vi "Keyboard Input with Sensitivity Support.vi"(2 "device ID":refnum<k1>, 3 "Previous Control Cluster":T1 {"Yaw Speed" scale=-1.0..1.0; "Vertical Speed" scale=-1.0..1.0; "Pitch" scale=-1.0..1.0; "Roll" scale=-1.0..1.0}, 4 "Speed step":dbl, 5 "error in (no error)":errorcluster) -> (0 "error out":errorcluster, 1 "Control Cluster":T2 {"Roll" scale=-1.0..1.0; "Pitch" scale=-1.0..1.0; "Vertical Speed" scale=-1.0..1.0; "Yaw Speed" scale=-1.0..1.0})   [LabVIEW 2014]
uses:
  <vilib>/Utility/inputDevices.llb/keyboardAcquire.vi
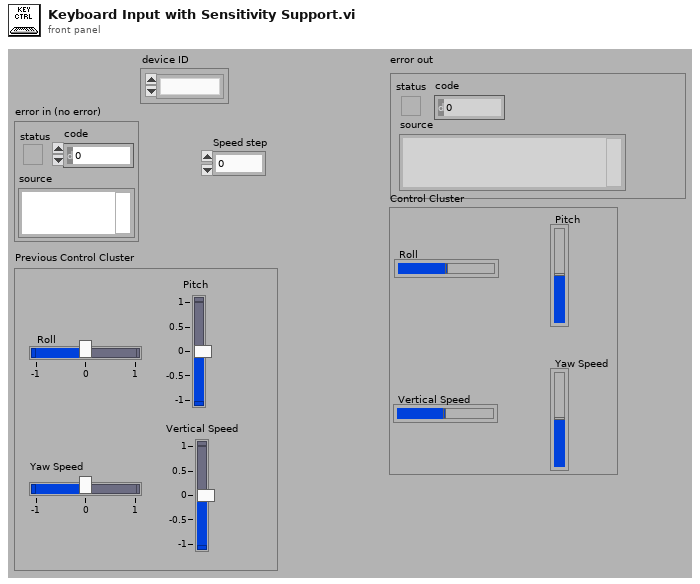
[diagram p1: front panel]
types:
  T1 = cluster{"Roll":sgl, "Pitch":sgl, "Vertical Speed":sgl, "Yaw Speed":sgl}
  T2 = cluster{"Roll":dbl, "Pitch":dbl, "Vertical Speed":dbl, "Yaw Speed":dbl}
  T3 = enum16{"0", "1", "2", "3", "4", "5", "6", "7", "8", "9", "A", "B", "C", "D", "E", "F", "G", "H", "I", "J", "K", "L", "M", "N", "O", "P", "Q", "R", "S", "T", "U", "V", "W", "X", "Y", "Z", "F1", "F2", "F3", "F4", "F5", "F6", "F7", "F8", "F9", "F10", "F11", "F12", "F13", "F14", "F15", "ADD", "BACK", "BACKSLASH", "CAPITAL", "COMMA", "DECIMAL", "DELETE", "DIVIDE", "DOWN", "END", "EQUALS", "ESCAPE", "GRAVE (`)", "HOME", "INSERT", "LBRACKET", "LCONTROL", "LEFT", "L ALT", "LSHIFT", "LWIN", "MINUS", "MULTIPLY", "NEXT", "NUMLOCK", "NUMPAD_0", "NUMPAD_1", "NUMPAD_2", "NUMPAD_3", "NUMPAD_4", "NUMPAD_5", "NUMPAD_6", "NUMPAD_7", "NUMPAD_8", "NUMPAD_9", "PAUSE", "PERIOD", "PRIOR (PG UP)", "RBRACKET", "RCONTROL", "RETURN", "RIGHT", "R ALT", "RSHIFT", "RWIN", "SCROLL", "SEMICOLON", "SLASH", "SPACE", "SUBTRACT", "TAB", "UP", "ENTER (num pad)", "' (quote)"}[]
  T4 = enum16{"0", "1", "2", "3", "4", "5", "6", "7", "8", "9", "A", "B", "C", "D", "E", "F", "G", "H", "I", "J", "K", "L", "M", "N", "O", "P", "Q", "R", "S", "T", "U", "V", "W", "X", "Y", "Z", "F1", "F2", "F3", "F4", "F5", "F6", "F7", "F8", "F9", "F10", "F11", "F12", "F13", "F14", "F15", "ADD", "BACK", "BACKSLASH", "CAPITAL", "COMMA", "DECIMAL", "DELETE", "DIVIDE", "DOWN", "END", "EQUALS", "ESCAPE", "GRAVE (`)", "HOME", "INSERT", "LBRACKET", "LCONTROL", "LEFT", "L ALT", "LSHIFT", "LWIN", "MINUS", "MULTIPLY", "NEXT", "NUMLOCK", "NUMPAD_0", "NUMPAD_1", "NUMPAD_2", "NUMPAD_3", "NUMPAD_4", "NUMPAD_5", "NUMPAD_6", "NUMPAD_7", "NUMPAD_8", "NUMPAD_9", "PAUSE", "PERIOD", "PRIOR (PG UP)", "RBRACKET", "RCONTROL", "RETURN", "RIGHT", "R ALT", "RSHIFT", "RWIN", "SCROLL", "SEMICOLON", "SLASH", "SPACE", "SUBTRACT", "TAB", "UP", "ENTER (num pad)", "' (quote)"}
  T5 = cluster{dbl, dbl, "New Speed":dbl, "New Speed":dbl}
  T6 = cluster{dbl, "New Speed":dbl, "New Speed":dbl, dbl}
  T7 = cluster{"New Speed":dbl, dbl, "New Speed":dbl, dbl}
  T8 = cluster{dbl, "New Speed":dbl, dbl, "New Speed":dbl}
  T9 = cluster{"New Speed":dbl, dbl, dbl, "New Speed":dbl}
  T10 = cluster{"New Speed":dbl, "New Speed":dbl, dbl, dbl}
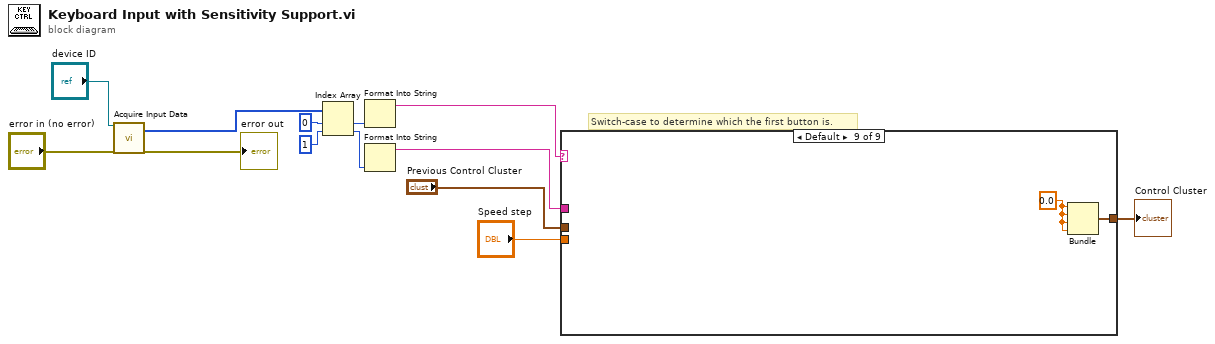
[diagram p0: block diagram]
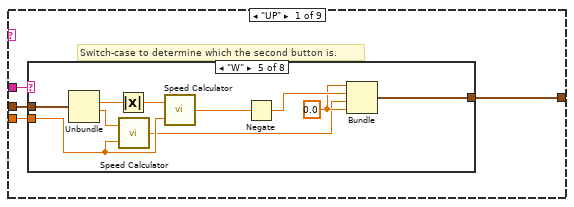
[diagram p2: hidden frame]
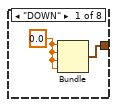
[diagram p3: hidden frame]
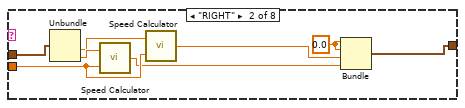
[diagram p4: hidden frame]
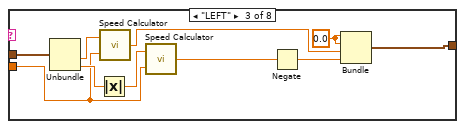
[diagram p5: hidden frame]
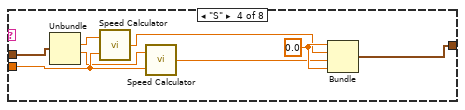
[diagram p6: hidden frame]
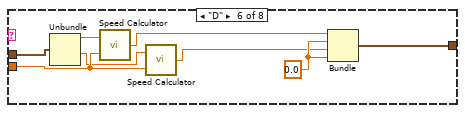
[diagram p7: hidden frame]
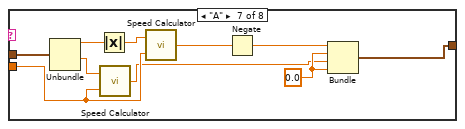
[diagram p8: hidden frame]
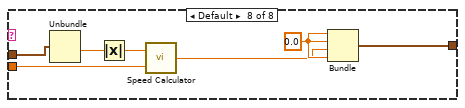
[diagram p9: hidden frame]
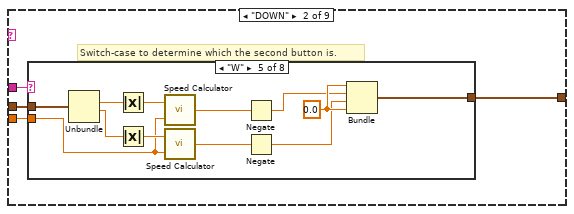
[diagram p10: hidden frame]
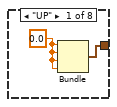
[diagram p11: hidden frame]
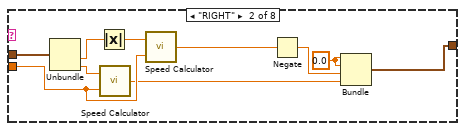
[diagram p12: hidden frame]
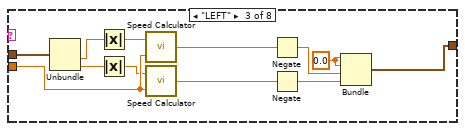
[diagram p13: hidden frame]
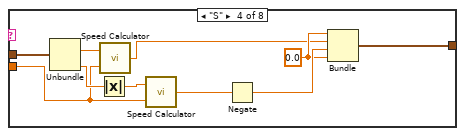
[diagram p14: hidden frame]
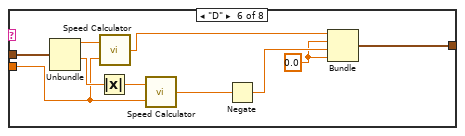
[diagram p15: hidden frame]
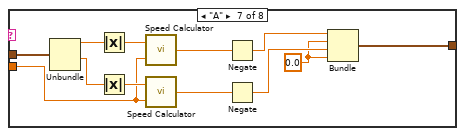
[diagram p16: hidden frame]
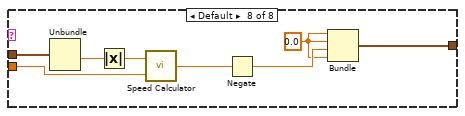
[diagram p17: hidden frame]
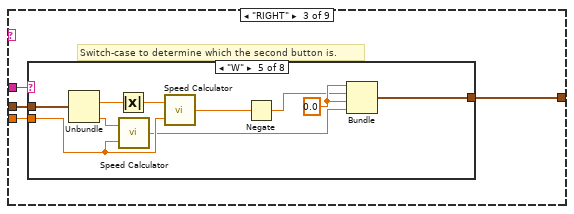
[diagram p18: hidden frame]
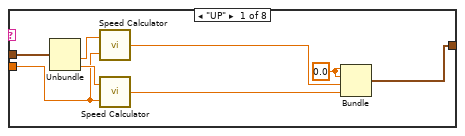
[diagram p19: hidden frame]
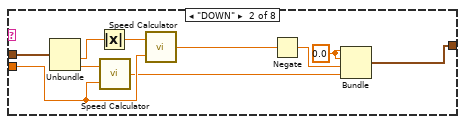
[diagram p20: hidden frame]
diagram:
  # "Switch-case to determine which the first button is."
  n1 = call-poly <vilib>:"Acquire Input Data.vi"("device ID"="device ID", "error in (no error)"="error in (no error)") -> ("keys pressed"=w7:T3, "error out"=→"error out":errorcluster)  [unwired: 15 in, 1 out]
  n2 = Index Array(array=w7, index #1=0, index #2=1) -> (element #1=w11:T4, element #2=w5:T4)
  n3 = Format Into String(w11) -> (resulting string=w13:string)  [unwired: 3 in, 1 out]
  n4 = Format Into String(w5) -> (resulting string=w4:string)  [unwired: 3 in, 1 out]
  n5 = case shown="Default" w13 {
    tunnel: w4 -> [w17 w83 w163 w230 w309 w375 w455 w521 _]
    tunnel: [w16 w82 w162 w228 w308 w374 w454 w520 w599] -> w2
    tunnel: "Speed step" -> [w15 w84 w164 w229 w310 w376 w456 w522 _]
    tunnel: "Previous Control Cluster" -> [w14 w81 w161 w227 w307 w373 w453 w519 _]
    frame "UP" {
      # "Switch-case to determine which the second button is."
      n6 = case shown="\"W\"" w17 {
        tunnel: [w18 w26 w37 w45 w55 w63 w73 w79] -> w16
        tunnel: w15 -> [_ w22 w31 w42 w49 w59 w68 w78]
        tunnel: w14 -> [_ w25 w34 w43 w52 w61 w70 w76]
        frame "DOWN" {
          w19 = 0.0
          n7 = Bundle(w19, w19, w19, w19) -> (w18:cluster{dbl, dbl, dbl, dbl})  [unwired: 1 in]
        }
        frame "RIGHT" {
          w27 = 0.0
          n8 = Unbundle(w25) -> ("Vertical Speed"=w20:sgl, "Yaw Speed"=w23:sgl)  [unwired: 2 out]
          n9 = call "Speed Calculator.vi"("Speed step"=w22, "Previous Speed"=w23) -> ("New Speed"=w21:dbl)
          n10 = call "Speed Calculator.vi"("Speed step"=w22, "Previous Speed"=w20) -> ("New Speed"=w24:dbl)
          n11 = Bundle(w27, w27, "New Speed"=w24, "New Speed"=w21) -> (w26:T5)  [unwired: 1 in]
        }
        frame "LEFT" {
          w35 = 0.0
          n12 = Unbundle(w34) -> ("Vertical Speed"=w30:sgl, "Yaw Speed"=w33:sgl)  [unwired: 2 out]
          n13 = Absolute Value(x=w33) -> (abs(x)=w32:sgl)
          n14 = call "Speed Calculator.vi"("Speed step"=w31, "Previous Speed"=w30) -> ("New Speed"=w29:dbl)
          n15 = call "Speed Calculator.vi"("Speed step"=w31, "Previous Speed"=w32) -> ("New Speed"=w28:dbl)
          n16 = Negate(x=w28) -> (-x=w36:dbl)
          n17 = Bundle(w35, w35, "New Speed"=w29, w36) -> (w37:cluster{dbl, dbl, "New Speed":dbl, dbl})  [unwired: 1 in]
        }
        frame "S" {
          w44 = 0.0
          n18 = Unbundle(w43) -> ("Pitch"=w38:sgl, "Vertical Speed"=w41:sgl)  [unwired: 2 out]
          n19 = call "Speed Calculator.vi"("Speed step"=w42, "Previous Speed"=w38) -> ("New Speed"=w39:dbl)
          n20 = call "Speed Calculator.vi"("Speed step"=w42, "Previous Speed"=w41) -> ("New Speed"=w40:dbl)
          n21 = Bundle(w44, "New Speed"=w39, "New Speed"=w40, w44) -> (w45:T6)  [unwired: 1 in]
        }
        frame "W" {
          w53 = 0.0
          n22 = Unbundle(w52) -> ("Pitch"=w51:sgl, "Vertical Speed"=w48:sgl)  [unwired: 2 out]
          n23 = Absolute Value(x=w51) -> (abs(x)=w50:sgl)
          n24 = call "Speed Calculator.vi"("Speed step"=w49, "Previous Speed"=w48) -> ("New Speed"=w47:dbl)
          n25 = call "Speed Calculator.vi"("Speed step"=w49, "Previous Speed"=w50) -> ("New Speed"=w46:dbl)
          n26 = Negate(x=w46) -> (-x=w54:dbl)
          n27 = Bundle(w53, w54, "New Speed"=w47, w53) -> (w55:cluster{dbl, dbl, "New Speed":dbl, dbl})  [unwired: 1 in]
        }
        frame "D" {
          w62 = 0.0
          n28 = Unbundle(w61) -> ("Roll"=w60:sgl, "Vertical Speed"=w58:sgl)  [unwired: 2 out]
          n29 = call "Speed Calculator.vi"("Speed step"=w59, "Previous Speed"=w60) -> ("New Speed"=w56:dbl)
          n30 = call "Speed Calculator.vi"("Speed step"=w59, "Previous Speed"=w58) -> ("New Speed"=w57:dbl)
          n31 = Bundle("New Speed"=w56, w62, "New Speed"=w57, w62) -> (w63:T7)  [unwired: 1 in]
        }
        frame "A" {
          w71 = 0.0
          n32 = Unbundle(w70) -> ("Roll"=w66:sgl, "Vertical Speed"=w69:sgl)  [unwired: 2 out]
          n33 = Absolute Value(x=w66) -> (abs(x)=w67:sgl)
          n34 = call "Speed Calculator.vi"("Speed step"=w68, "Previous Speed"=w69) -> ("New Speed"=w64:dbl)
          n35 = call "Speed Calculator.vi"("Speed step"=w68, "Previous Speed"=w67) -> ("New Speed"=w65:dbl)
          n36 = Negate(x=w65) -> (-x=w72:dbl)
          n37 = Bundle(w72, w71, "New Speed"=w64, w71) -> (w73:cluster{dbl, dbl, "New Speed":dbl, dbl})  [unwired: 1 in]
        }
        frame Default {
          w80 = 0.0
          n38 = Unbundle(w76) -> ("Vertical Speed"=w75:sgl)  [unwired: 3 out]
          n39 = Absolute Value(x=w75) -> (abs(x)=w74:sgl)
          n40 = call "Speed Calculator.vi"("Speed step"=w78, "Previous Speed"=w74) -> ("New Speed"=w77:dbl)
          n41 = Bundle(w80, w80, "New Speed"=w77, w80) -> (w79:cluster{dbl, dbl, "New Speed":dbl, dbl})  [unwired: 1 in]
        }
      }
    }
    frame "DOWN" {
      # "Switch-case to determine which the second button is."
      n42 = case shown="\"W\"" w83 {
        tunnel: [w86 w95 w108 w117 w130 w139 w152 w158] -> w82
        tunnel: w84 -> [_ w90 w103 w112 w123 w133 w141 w154]
        tunnel: w81 -> [_ w93 w106 w115 w128 w137 w148 w157]
        frame "UP" {
          w85 = 0.0
          n43 = Bundle(w85, w85, w85, w85) -> (w86:cluster{dbl, dbl, dbl, dbl})  [unwired: 1 in]
        }
        frame "RIGHT" {
          w94 = 0.0
          n44 = Unbundle(w93) -> ("Vertical Speed"=w92:sgl, "Yaw Speed"=w89:sgl)  [unwired: 2 out]
          n45 = Absolute Value(x=w92) -> (abs(x)=w91:sgl)
          n46 = call "Speed Calculator.vi"("Speed step"=w90, "Previous Speed"=w89) -> ("New Speed"=w88:dbl)
          n47 = call "Speed Calculator.vi"("Speed step"=w90, "Previous Speed"=w91) -> ("New Speed"=w87:dbl)
          n48 = Negate(x=w87) -> (-x=w96:dbl)
          n49 = Bundle(w94, w94, w96, "New Speed"=w88) -> (w95:cluster{dbl, dbl, dbl, "New Speed":dbl})  [unwired: 1 in]
        }
        frame "LEFT" {
          w107 = 0.0
          n50 = Unbundle(w106) -> ("Vertical Speed"=w105:sgl, "Yaw Speed"=w101:sgl)  [unwired: 2 out]
          n51 = Absolute Value(x=w105) -> (abs(x)=w104:sgl)
          n52 = Absolute Value(x=w101) -> (abs(x)=w102:sgl)
          n53 = call "Speed Calculator.vi"("Speed step"=w103, "Previous Speed"=w104) -> ("New Speed"=w100:dbl)
          n54 = call "Speed Calculator.vi"("Speed step"=w103, "Previous Speed"=w102) -> ("New Speed"=w99:dbl)
          n55 = Negate(x=w100) -> (-x=w98:dbl)
          n56 = Negate(x=w99) -> (-x=w97:dbl)
          n57 = Bundle(w107, w107, w98, w97) -> (w108:cluster{dbl, dbl, dbl, dbl})  [unwired: 1 in]
        }
        frame "S" {
          w116 = 0.0
          n58 = Unbundle(w115) -> ("Pitch"=w111:sgl, "Yaw Speed"=w114:sgl)  [unwired: 2 out]
          n59 = Absolute Value(x=w114) -> (abs(x)=w113:sgl)
          n60 = call "Speed Calculator.vi"("Speed step"=w112, "Previous Speed"=w111) -> ("New Speed"=w110:dbl)
          n61 = call "Speed Calculator.vi"("Speed step"=w112, "Previous Speed"=w113) -> ("New Speed"=w109:dbl)
          n62 = Negate(x=w109) -> (-x=w118:dbl)
          n63 = Bundle(w116, "New Speed"=w110, w118, w116) -> (w117:cluster{dbl, "New Speed":dbl, dbl, dbl})  [unwired: 1 in]
        }
        frame "W" {
          w129 = 0.0
          n64 = Unbundle(w128) -> ("Pitch"=w127:sgl, "Vertical Speed"=w125:sgl)  [unwired: 2 out]
          n65 = Absolute Value(x=w127) -> (abs(x)=w126:sgl)
          n66 = Absolute Value(x=w125) -> (abs(x)=w124:sgl)
          n67 = call "Speed Calculator.vi"("Speed step"=w123, "Previous Speed"=w126) -> ("New Speed"=w122:dbl)
          n68 = call "Speed Calculator.vi"("Speed step"=w123, "Previous Speed"=w124) -> ("New Speed"=w121:dbl)
          n69 = Negate(x=w122) -> (-x=w120:dbl)
          n70 = Negate(x=w121) -> (-x=w119:dbl)
          n71 = Bundle(w129, w120, w119, w129) -> (w130:cluster{dbl, dbl, dbl, dbl})  [unwired: 1 in]
        }
        frame "D" {
          w138 = 0.0
          n72 = Unbundle(w137) -> ("Roll"=w131:sgl, "Vertical Speed"=w136:sgl)  [unwired: 2 out]
          n73 = Absolute Value(x=w136) -> (abs(x)=w135:sgl)
          n74 = call "Speed Calculator.vi"("Speed step"=w133, "Previous Speed"=w131) -> ("New Speed"=w132:dbl)
          n75 = call "Speed Calculator.vi"("Speed step"=w133, "Previous Speed"=w135) -> ("New Speed"=w134:dbl)
          n76 = Negate(x=w134) -> (-x=w140:dbl)
          n77 = Bundle("New Speed"=w132, w138, w140, w138) -> (w139:cluster{"New Speed":dbl, dbl, dbl, dbl})  [unwired: 1 in]
        }
        frame "A" {
          w150 = 0.0
          n78 = Unbundle(w148) -> ("Roll"=w147:sgl, "Vertical Speed"=w145:sgl)  [unwired: 2 out]
          n79 = Absolute Value(x=w147) -> (abs(x)=w146:sgl)
          n80 = Absolute Value(x=w145) -> (abs(x)=w144:sgl)
          n81 = call "Speed Calculator.vi"("Speed step"=w141, "Previous Speed"=w146) -> ("New Speed"=w142:dbl)
          n82 = call "Speed Calculator.vi"("Speed step"=w141, "Previous Speed"=w144) -> ("New Speed"=w143:dbl)
          n83 = Negate(x=w142) -> (-x=w149:dbl)
          n84 = Negate(x=w143) -> (-x=w151:dbl)
          n85 = Bundle(w149, w150, w151, w150) -> (w152:cluster{dbl, dbl, dbl, dbl})  [unwired: 1 in]
        }
        frame Default {
          w159 = 0.0
          n86 = Unbundle(w157) -> ("Vertical Speed"=w153:sgl)  [unwired: 3 out]
          n87 = Absolute Value(x=w153) -> (abs(x)=w156:sgl)
          n88 = call "Speed Calculator.vi"("Speed step"=w154, "Previous Speed"=w156) -> ("New Speed"=w155:dbl)
          n89 = Negate(x=w155) -> (-x=w160:dbl)
          n90 = Bundle(w159, w159, w160, w159) -> (w158:cluster{dbl, dbl, dbl, dbl})  [unwired: 1 in]
        }
      }
    }
    frame "RIGHT" {
      # "Switch-case to determine which the second button is."
      n91 = case shown="\"W\"" w163 {
        tunnel: [w171 w180 w183 w192 w202 w210 w220 w225] -> w162
        tunnel: w164 -> [w167 w175 _ w187 w195 w205 w211 w221]
        tunnel: w161 -> [w170 w179 _ w190 w199 w208 w217 w224]
        frame "UP" {
          w172 = 0.0
          n92 = Unbundle(w170) -> ("Vertical Speed"=w169:sgl, "Yaw Speed"=w168:sgl)  [unwired: 2 out]
          n93 = call "Speed Calculator.vi"("Speed step"=w167, "Previous Speed"=w169) -> ("New Speed"=w166:dbl)
          n94 = call "Speed Calculator.vi"("Speed step"=w167, "Previous Speed"=w168) -> ("New Speed"=w165:dbl)
          n95 = Bundle(w172, w172, "New Speed"=w166, "New Speed"=w165) -> (w171:T5)  [unwired: 1 in]
        }
        frame "DOWN" {
          w181 = 0.0
          n96 = Unbundle(w179) -> ("Vertical Speed"=w178:sgl, "Yaw Speed"=w174:sgl)  [unwired: 2 out]
          n97 = Absolute Value(x=w178) -> (abs(x)=w177:sgl)
          n98 = call "Speed Calculator.vi"("Speed step"=w175, "Previous Speed"=w174) -> ("New Speed"=w173:dbl)
          n99 = call "Speed Calculator.vi"("Speed step"=w175, "Previous Speed"=w177) -> ("New Speed"=w176:dbl)
          n100 = Negate(x=w176) -> (-x=w182:dbl)
          n101 = Bundle(w181, w181, w182, "New Speed"=w173) -> (w180:cluster{dbl, dbl, dbl, "New Speed":dbl})  [unwired: 1 in]
        }
        frame "LEFT" {
          w184 = 0.0
          n102 = Bundle(w184, w184, w184, w184) -> (w183:cluster{dbl, dbl, dbl, dbl})  [unwired: 1 in]
        }
        frame "S" {
          w191 = 0.0
          n103 = Unbundle(w190) -> ("Pitch"=w189:sgl, "Yaw Speed"=w188:sgl)  [unwired: 2 out]
          n104 = call "Speed Calculator.vi"("Speed step"=w187, "Previous Speed"=w189) -> ("New Speed"=w186:dbl)
          n105 = call "Speed Calculator.vi"("Speed step"=w187, "Previous Speed"=w188) -> ("New Speed"=w185:dbl)
          n106 = Bundle(w191, "New Speed"=w186, w191, "New Speed"=w185) -> (w192:T8)  [unwired: 1 in]
        }
        frame "W" {
          w201 = 0.0
          n107 = Unbundle(w199) -> ("Pitch"=w198:sgl, "Yaw Speed"=w194:sgl)  [unwired: 2 out]
          n108 = Absolute Value(x=w198) -> (abs(x)=w197:sgl)
          n109 = call "Speed Calculator.vi"("Speed step"=w195, "Previous Speed"=w194) -> ("New Speed"=w193:dbl)
          n110 = call "Speed Calculator.vi"("Speed step"=w195, "Previous Speed"=w197) -> ("New Speed"=w196:dbl)
          n111 = Negate(x=w196) -> (-x=w200:dbl)
          n112 = Bundle(w201, w200, w201, "New Speed"=w193) -> (w202:cluster{dbl, dbl, dbl, "New Speed":dbl})  [unwired: 1 in]
        }
        frame "D" {
          w209 = 0.0
          n113 = Unbundle(w208) -> ("Roll"=w207:sgl, "Yaw Speed"=w206:sgl)  [unwired: 2 out]
          n114 = call "Speed Calculator.vi"("Speed step"=w205, "Previous Speed"=w207) -> ("New Speed"=w204:dbl)
          n115 = call "Speed Calculator.vi"("Speed step"=w205, "Previous Speed"=w206) -> ("New Speed"=w203:dbl)
          n116 = Bundle("New Speed"=w204, w209, w209, "New Speed"=w203) -> (w210:T9)  [unwired: 1 in]
        }
        frame "A" {
          w218 = 0.0
          n117 = Unbundle(w217) -> ("Roll"=w216:sgl, "Yaw Speed"=w213:sgl)  [unwired: 2 out]
          n118 = Absolute Value(x=w216) -> (abs(x)=w215:sgl)
          n119 = call "Speed Calculator.vi"("Speed step"=w211, "Previous Speed"=w213) -> ("New Speed"=w212:dbl)
          n120 = call "Speed Calculator.vi"("Speed step"=w211, "Previous Speed"=w215) -> ("New Speed"=w214:dbl)
          n121 = Negate(x=w214) -> (-x=w219:dbl)
          n122 = Bundle(w219, w218, w218, "New Speed"=w212) -> (w220:cluster{dbl, dbl, dbl, "New Speed":dbl})  [unwired: 1 in]
        }
        frame Default {
          w226 = 0.0
          n123 = Unbundle(w224) -> ("Yaw Speed"=w223:sgl)  [unwired: 3 out]
          n124 = call "Speed Calculator.vi"("Speed step"=w221, "Previous Speed"=w223) -> ("New Speed"=w222:dbl)
          n125 = Bundle(w226, w226, w226, "New Speed"=w222) -> (w225:cluster{dbl, dbl, dbl, "New Speed":dbl})  [unwired: 1 in]
        }
      }
    }
    frame "LEFT" {
      # "Switch-case to determine which the second button is."
      n126 = case shown="\"W\"" w230 {
        tunnel: [w238 w250 w253 w263 w276 w285 w298 w306] -> w228
        tunnel: w229 -> [w231 w241 _ w255 w265 w277 w291 w299]
        tunnel: w227 -> [w237 w249 _ w261 w274 w283 w296 w303]
        frame "UP" {
          w239 = 0.0
          n127 = Unbundle(w237) -> ("Vertical Speed"=w232:sgl, "Yaw Speed"=w236:sgl)  [unwired: 2 out]
          n128 = Absolute Value(x=w236) -> (abs(x)=w235:sgl)
          n129 = call "Speed Calculator.vi"("Speed step"=w231, "Previous Speed"=w232) -> ("New Speed"=w233:dbl)
          n130 = call "Speed Calculator.vi"("Speed step"=w231, "Previous Speed"=w235) -> ("New Speed"=w234:dbl)
          n131 = Negate(x=w234) -> (-x=w240:dbl)
          n132 = Bundle(w239, w239, "New Speed"=w233, w240) -> (w238:cluster{dbl, dbl, "New Speed":dbl, dbl})  [unwired: 1 in]
        }
        frame "DOWN" {
          w251 = 0.0
          n133 = Unbundle(w249) -> ("Vertical Speed"=w243:sgl, "Yaw Speed"=w242:sgl)  [unwired: 2 out]
          n134 = Absolute Value(x=w243) -> (abs(x)=w245:sgl)
          n135 = Absolute Value(x=w242) -> (abs(x)=w244:sgl)
          n136 = call "Speed Calculator.vi"("Speed step"=w241, "Previous Speed"=w245) -> ("New Speed"=w247:dbl)
          n137 = call "Speed Calculator.vi"("Speed step"=w241, "Previous Speed"=w244) -> ("New Speed"=w246:dbl)
          n138 = Negate(x=w247) -> (-x=w248:dbl)
          n139 = Negate(x=w246) -> (-x=w252:dbl)
          n140 = Bundle(w251, w251, w248, w252) -> (w250:cluster{dbl, dbl, dbl, dbl})  [unwired: 1 in]
        }
        frame "RIGHT" {
          w254 = 0.0
          n141 = Bundle(w254, w254, w254, w254) -> (w253:cluster{dbl, dbl, dbl, dbl})  [unwired: 1 in]
        }
        frame "S" {
          w262 = 0.0
          n142 = Unbundle(w261) -> ("Pitch"=w260:sgl, "Yaw Speed"=w258:sgl)  [unwired: 2 out]
          n143 = Absolute Value(x=w258) -> (abs(x)=w257:sgl)
          n144 = call "Speed Calculator.vi"("Speed step"=w255, "Previous Speed"=w260) -> ("New Speed"=w259:dbl)
          n145 = call "Speed Calculator.vi"("Speed step"=w255, "Previous Speed"=w257) -> ("New Speed"=w256:dbl)
          n146 = Negate(x=w256) -> (-x=w264:dbl)
          n147 = Bundle(w262, "New Speed"=w259, w262, w264) -> (w263:cluster{dbl, "New Speed":dbl, dbl, dbl})  [unwired: 1 in]
        }
        frame "W" {
          w275 = 0.0
          n148 = Unbundle(w274) -> ("Pitch"=w273:sgl, "Yaw Speed"=w272:sgl)  [unwired: 2 out]
          n149 = Absolute Value(x=w273) -> (abs(x)=w270:sgl)
          n150 = Absolute Value(x=w272) -> (abs(x)=w271:sgl)
          n151 = call "Speed Calculator.vi"("Speed step"=w265, "Previous Speed"=w270) -> ("New Speed"=w269:dbl)
          n152 = call "Speed Calculator.vi"("Speed step"=w265, "Previous Speed"=w271) -> ("New Speed"=w268:dbl)
          n153 = Negate(x=w269) -> (-x=w267:dbl)
          n154 = Negate(x=w268) -> (-x=w266:dbl)
          n155 = Bundle(w275, w267, w275, w266) -> (w276:cluster{dbl, dbl, dbl, dbl})  [unwired: 1 in]
        }
        frame "D" {
          w284 = 0.0
          n156 = Unbundle(w283) -> ("Roll"=w282:sgl, "Yaw Speed"=w280:sgl)  [unwired: 2 out]
          n157 = Absolute Value(x=w280) -> (abs(x)=w279:sgl)
          n158 = call "Speed Calculator.vi"("Speed step"=w277, "Previous Speed"=w282) -> ("New Speed"=w281:dbl)
          n159 = call "Speed Calculator.vi"("Speed step"=w277, "Previous Speed"=w279) -> ("New Speed"=w278:dbl)
          n160 = Negate(x=w278) -> (-x=w286:dbl)
          n161 = Bundle("New Speed"=w281, w284, w284, w286) -> (w285:cluster{"New Speed":dbl, dbl, dbl, dbl})  [unwired: 1 in]
        }
        frame "A" {
          w297 = 0.0
          n162 = Unbundle(w296) -> ("Roll"=w295:sgl, "Yaw Speed"=w294:sgl)  [unwired: 2 out]
          n163 = Absolute Value(x=w295) -> (abs(x)=w293:sgl)
          n164 = Absolute Value(x=w294) -> (abs(x)=w292:sgl)
          n165 = call "Speed Calculator.vi"("Speed step"=w291, "Previous Speed"=w293) -> ("New Speed"=w290:dbl)
          n166 = call "Speed Calculator.vi"("Speed step"=w291, "Previous Speed"=w292) -> ("New Speed"=w289:dbl)
          n167 = Negate(x=w290) -> (-x=w288:dbl)
          n168 = Negate(x=w289) -> (-x=w287:dbl)
          n169 = Bundle(w288, w297, w297, w287) -> (w298:cluster{dbl, dbl, dbl, dbl})  [unwired: 1 in]
        }
        frame Default {
          w305 = 0.0
          n170 = Unbundle(w303) -> ("Yaw Speed"=w302:sgl)  [unwired: 3 out]
          n171 = Absolute Value(x=w302) -> (abs(x)=w301:sgl)
          n172 = call "Speed Calculator.vi"("Speed step"=w299, "Previous Speed"=w301) -> ("New Speed"=w300:dbl)
          n173 = Negate(x=w300) -> (-x=w304:dbl)
          n174 = Bundle(w305, w305, w305, w304) -> (w306:cluster{dbl, dbl, dbl, dbl})  [unwired: 1 in]
        }
      }
    }
    frame "S" {
      # "Switch-case to determine which the second button is."
      n175 = case shown="\"W\"" w309 {
        tunnel: [w318 w327 w336 w345 w347 w355 w365 w372] -> w308
        tunnel: w310 -> [w311 w319 w329 w337 _ w349 w357 w367]
        tunnel: w307 -> [w317 w325 w335 w344 _ w354 w363 w370]
        frame "UP" {
          w316 = 0.0
          n176 = Unbundle(w317) -> ("Pitch"=w315:sgl, "Vertical Speed"=w314:sgl)  [unwired: 2 out]
          n177 = call "Speed Calculator.vi"("Speed step"=w311, "Previous Speed"=w315) -> ("New Speed"=w313:dbl)
          n178 = call "Speed Calculator.vi"("Speed step"=w311, "Previous Speed"=w314) -> ("New Speed"=w312:dbl)
          n179 = Bundle(w316, "New Speed"=w313, "New Speed"=w312, w316) -> (w318:T6)  [unwired: 1 in]
        }
        frame "DOWN" {
          w326 = 0.0
          n180 = Unbundle(w325) -> ("Pitch"=w324:sgl, "Vertical Speed"=w323:sgl)  [unwired: 2 out]
          n181 = Absolute Value(x=w323) -> (abs(x)=w322:sgl)
          n182 = call "Speed Calculator.vi"("Speed step"=w319, "Previous Speed"=w324) -> ("New Speed"=w320:dbl)
          n183 = call "Speed Calculator.vi"("Speed step"=w319, "Previous Speed"=w322) -> ("New Speed"=w321:dbl)
          n184 = Negate(x=w321) -> (-x=w328:dbl)
          n185 = Bundle(w326, "New Speed"=w320, w328, w326) -> (w327:cluster{dbl, "New Speed":dbl, dbl, dbl})  [unwired: 1 in]
        }
        frame "RIGHT" {
          w334 = 0.0
          n186 = Unbundle(w335) -> ("Pitch"=w333:sgl, "Vertical Speed"=w330:sgl)  [unwired: 2 out]
          n187 = call "Speed Calculator.vi"("Speed step"=w329, "Previous Speed"=w333) -> ("New Speed"=w332:dbl)
          n188 = call "Speed Calculator.vi"("Speed step"=w329, "Previous Speed"=w330) -> ("New Speed"=w331:dbl)
          n189 = Bundle(w334, "New Speed"=w332, w334, "New Speed"=w331) -> (w336:T8)  [unwired: 1 in]
        }
        frame "LEFT" {
          w343 = 0.0
          n190 = Unbundle(w344) -> ("Pitch"=w338:sgl, "Yaw Speed"=w342:sgl)  [unwired: 2 out]
          n191 = Absolute Value(x=w342) -> (abs(x)=w341:sgl)
          n192 = call "Speed Calculator.vi"("Speed step"=w337, "Previous Speed"=w338) -> ("New Speed"=w339:dbl)
          n193 = call "Speed Calculator.vi"("Speed step"=w337, "Previous Speed"=w341) -> ("New Speed"=w340:dbl)
          n194 = Negate(x=w340) -> (-x=w346:dbl)
          n195 = Bundle(w343, "New Speed"=w339, w343, w346) -> (w345:cluster{dbl, "New Speed":dbl, dbl, dbl})  [unwired: 1 in]
        }
        frame "W" {
          w348 = 0.0
          n196 = Bundle(w348, w348, w348, w348) -> (w347:cluster{dbl, dbl, dbl, dbl})  [unwired: 1 in]
        }
        frame "D" {
          w356 = 0.0
          n197 = Unbundle(w354) -> ("Roll"=w353:sgl, "Pitch"=w351:sgl)  [unwired: 2 out]
          n198 = call "Speed Calculator.vi"("Speed step"=w349, "Previous Speed"=w353) -> ("New Speed"=w352:dbl)
          n199 = call "Speed Calculator.vi"("Speed step"=w349, "Previous Speed"=w351) -> ("New Speed"=w350:dbl)
          n200 = Bundle("New Speed"=w352, "New Speed"=w350, w356, w356) -> (w355:T10)  [unwired: 1 in]
        }
        frame "A" {
          w366 = 0.0
          n201 = Unbundle(w363) -> ("Roll"=w362:sgl, "Pitch"=w359:sgl)  [unwired: 2 out]
          n202 = Absolute Value(x=w362) -> (abs(x)=w361:sgl)
          n203 = call "Speed Calculator.vi"("Speed step"=w357, "Previous Speed"=w359) -> ("New Speed"=w358:dbl)
          n204 = call "Speed Calculator.vi"("Speed step"=w357, "Previous Speed"=w361) -> ("New Speed"=w360:dbl)
          n205 = Negate(x=w360) -> (-x=w364:dbl)
          n206 = Bundle(w364, "New Speed"=w358, w366, w366) -> (w365:cluster{dbl, "New Speed":dbl, dbl, dbl})  [unwired: 1 in]
        }
        frame Default {
          w371 = 0.0
          n207 = Unbundle(w370) -> ("Pitch"=w369:sgl)  [unwired: 3 out]
          n208 = call "Speed Calculator.vi"("Speed step"=w367, "Previous Speed"=w369) -> ("New Speed"=w368:dbl)
          n209 = Bundle(w371, "New Speed"=w368, w371, w371) -> (w372:cluster{dbl, "New Speed":dbl, dbl, dbl})  [unwired: 1 in]
        }
      }
    }
    frame "W" {
      # "Switch-case to determine which the second button is."
      n210 = case shown="\"S\"" w375 {
        tunnel: [w386 w397 w408 w420 w421 w431 w442 w452] -> w374
        tunnel: w376 -> [w381 w389 w401 w411 _ w425 w433 w446]
        tunnel: w373 -> [w385 w396 w407 w416 _ w429 w436 w449]
        frame "UP" {
          w377 = 0.0
          n211 = Unbundle(w385) -> ("Roll"=w384:sgl, "Vertical Speed"=w380:sgl)  [unwired: 2 out]
          n212 = Absolute Value(x=w384) -> (abs(x)=w383:sgl)
          n213 = call "Speed Calculator.vi"("Speed step"=w381, "Previous Speed"=w380) -> ("New Speed"=w379:dbl)
          n214 = call "Speed Calculator.vi"("Speed step"=w381, "Previous Speed"=w383) -> ("New Speed"=w382:dbl)
          n215 = Negate(x=w382) -> (-x=w378:dbl)
          n216 = Bundle(w377, w378, "New Speed"=w379, w377) -> (w386:cluster{dbl, dbl, "New Speed":dbl, dbl})  [unwired: 1 in]
        }
        frame "DOWN" {
          w388 = 0.0
          n217 = Unbundle(w396) -> ("Roll"=w395:sgl, "Vertical Speed"=w391:sgl)  [unwired: 2 out]
          n218 = Absolute Value(x=w395) -> (abs(x)=w394:sgl)
          n219 = Absolute Value(x=w391) -> (abs(x)=w392:sgl)
          n220 = call "Speed Calculator.vi"("Speed step"=w389, "Previous Speed"=w394) -> ("New Speed"=w393:dbl)
          n221 = call "Speed Calculator.vi"("Speed step"=w389, "Previous Speed"=w392) -> ("New Speed"=w390:dbl)
          n222 = Negate(x=w393) -> (-x=w387:dbl)
          n223 = Negate(x=w390) -> (-x=w398:dbl)
          n224 = Bundle(w388, w387, w398, w388) -> (w397:cluster{dbl, dbl, dbl, dbl})  [unwired: 1 in]
        }
        frame "RIGHT" {
          w400 = 0.0
          n225 = Unbundle(w407) -> ("Roll"=w406:sgl, "Yaw Speed"=w404:sgl)  [unwired: 2 out]
          n226 = Absolute Value(x=w406) -> (abs(x)=w405:sgl)
          n227 = call "Speed Calculator.vi"("Speed step"=w401, "Previous Speed"=w404) -> ("New Speed"=w403:dbl)
          n228 = call "Speed Calculator.vi"("Speed step"=w401, "Previous Speed"=w405) -> ("New Speed"=w402:dbl)
          n229 = Negate(x=w402) -> (-x=w399:dbl)
          n230 = Bundle(w400, w399, w400, "New Speed"=w403) -> (w408:cluster{dbl, dbl, dbl, "New Speed":dbl})  [unwired: 1 in]
        }
        frame "LEFT" {
          w409 = 0.0
          n231 = Unbundle(w416) -> ("Roll"=w415:sgl, "Yaw Speed"=w413:sgl)  [unwired: 2 out]
          n232 = Absolute Value(x=w415) -> (abs(x)=w414:sgl)
          n233 = Absolute Value(x=w413) -> (abs(x)=w412:sgl)
          n234 = call "Speed Calculator.vi"("Speed step"=w411, "Previous Speed"=w414) -> ("New Speed"=w418:dbl)
          n235 = call "Speed Calculator.vi"("Speed step"=w411, "Previous Speed"=w412) -> ("New Speed"=w417:dbl)
          n236 = Negate(x=w418) -> (-x=w410:dbl)
          n237 = Negate(x=w417) -> (-x=w419:dbl)
          n238 = Bundle(w409, w410, w409, w419) -> (w420:cluster{dbl, dbl, dbl, dbl})  [unwired: 1 in]
        }
        frame "S" {
          w422 = 0.0
          n239 = Bundle(w422, w422, w422, w422) -> (w421:cluster{dbl, dbl, dbl, dbl})  [unwired: 1 in]
        }
        frame "D" {
          w432 = 0.0
          n240 = Unbundle(w429) -> ("Roll"=w424:sgl, "Pitch"=w428:sgl)  [unwired: 2 out]
          n241 = Absolute Value(x=w428) -> (abs(x)=w427:sgl)
          n242 = call "Speed Calculator.vi"("Speed step"=w425, "Previous Speed"=w424) -> ("New Speed"=w423:dbl)
          n243 = call "Speed Calculator.vi"("Speed step"=w425, "Previous Speed"=w427) -> ("New Speed"=w426:dbl)
          n244 = Negate(x=w426) -> (-x=w430:dbl)
          n245 = Bundle("New Speed"=w423, w430, w432, w432) -> (w431:cluster{"New Speed":dbl, dbl, dbl, dbl})  [unwired: 1 in]
        }
        frame "A" {
          w443 = 0.0
          n246 = Unbundle(w436) -> ("Roll"=w435:sgl, "Pitch"=w434:sgl)  [unwired: 2 out]
          n247 = Absolute Value(x=w435) -> (abs(x)=w438:sgl)
          n248 = Absolute Value(x=w434) -> (abs(x)=w437:sgl)
          n249 = call "Speed Calculator.vi"("Speed step"=w433, "Previous Speed"=w438) -> ("New Speed"=w440:dbl)
          n250 = call "Speed Calculator.vi"("Speed step"=w433, "Previous Speed"=w437) -> ("New Speed"=w439:dbl)
          n251 = Negate(x=w440) -> (-x=w441:dbl)
          n252 = Negate(x=w439) -> (-x=w444:dbl)
          n253 = Bundle(w441, w444, w443, w443) -> (w442:cluster{dbl, dbl, dbl, dbl})  [unwired: 1 in]
        }
        frame Default {
          w450 = 0.0
          n254 = Unbundle(w449) -> ("Pitch"=w445:sgl)  [unwired: 3 out]
          n255 = Absolute Value(x=w445) -> (abs(x)=w448:sgl)
          n256 = call "Speed Calculator.vi"("Speed step"=w446, "Previous Speed"=w448) -> ("New Speed"=w447:dbl)
          n257 = Negate(x=w447) -> (-x=w451:dbl)
          n258 = Bundle(w450, w451, w450, w450) -> (w452:cluster{dbl, dbl, dbl, dbl})  [unwired: 1 in]
        }
      }
    }
    frame "D" {
      # "Switch-case to determine which the second button is."
      n259 = case shown="\"W\"" w455 {
        tunnel: [w464 w473 w482 w491 w499 w509 w511 w518] -> w454
        tunnel: w456 -> [w458 w465 w475 w483 w493 w501 _ w513]
        tunnel: w453 -> [w462 w471 w480 w489 w498 w507 _ w516]
        frame "UP" {
          w463 = 0.0
          n260 = Unbundle(w462) -> ("Roll"=w461:sgl, "Vertical Speed"=w457:sgl)  [unwired: 2 out]
          n261 = call "Speed Calculator.vi"("Speed step"=w458, "Previous Speed"=w457) -> ("New Speed"=w459:dbl)
          n262 = call "Speed Calculator.vi"("Speed step"=w458, "Previous Speed"=w461) -> ("New Speed"=w460:dbl)
          n263 = Bundle("New Speed"=w460, w463, "New Speed"=w459, w463) -> (w464:T7)  [unwired: 1 in]
        }
        frame "DOWN" {
          w472 = 0.0
          n264 = Unbundle(w471) -> ("Roll"=w467:sgl, "Vertical Speed"=w470:sgl)  [unwired: 2 out]
          n265 = Absolute Value(x=w470) -> (abs(x)=w469:sgl)
          n266 = call "Speed Calculator.vi"("Speed step"=w465, "Previous Speed"=w467) -> ("New Speed"=w466:dbl)
          n267 = call "Speed Calculator.vi"("Speed step"=w465, "Previous Speed"=w469) -> ("New Speed"=w468:dbl)
          n268 = Negate(x=w468) -> (-x=w474:dbl)
          n269 = Bundle("New Speed"=w466, w472, w474, w472) -> (w473:cluster{"New Speed":dbl, dbl, dbl, dbl})  [unwired: 1 in]
        }
        frame "RIGHT" {
          w481 = 0.0
          n270 = Unbundle(w480) -> ("Roll"=w479:sgl, "Yaw Speed"=w478:sgl)  [unwired: 2 out]
          n271 = call "Speed Calculator.vi"("Speed step"=w475, "Previous Speed"=w479) -> ("New Speed"=w477:dbl)
          n272 = call "Speed Calculator.vi"("Speed step"=w475, "Previous Speed"=w478) -> ("New Speed"=w476:dbl)
          n273 = Bundle("New Speed"=w477, w481, w481, "New Speed"=w476) -> (w482:T9)  [unwired: 1 in]
        }
        frame "LEFT" {
          w490 = 0.0
          n274 = Unbundle(w489) -> ("Roll"=w485:sgl, "Yaw Speed"=w488:sgl)  [unwired: 2 out]
          n275 = Absolute Value(x=w488) -> (abs(x)=w487:sgl)
          n276 = call "Speed Calculator.vi"("Speed step"=w483, "Previous Speed"=w487) -> ("New Speed"=w486:dbl)
          n277 = Negate(x=w486) -> (-x=w492:dbl)
          n278 = call "Speed Calculator.vi"("Speed step"=w483, "Previous Speed"=w485) -> ("New Speed"=w484:dbl)
          n279 = Bundle("New Speed"=w484, w490, w490, w492) -> (w491:cluster{"New Speed":dbl, dbl, dbl, dbl})  [unwired: 1 in]
        }
        frame "S" {
          w500 = 0.0
          n280 = Unbundle(w498) -> ("Roll"=w497:sgl, "Pitch"=w496:sgl)  [unwired: 2 out]
          n281 = call "Speed Calculator.vi"("Speed step"=w493, "Previous Speed"=w497) -> ("New Speed"=w495:dbl)
          n282 = call "Speed Calculator.vi"("Speed step"=w493, "Previous Speed"=w496) -> ("New Speed"=w494:dbl)
          n283 = Bundle("New Speed"=w495, "New Speed"=w494, w500, w500) -> (w499:T10)  [unwired: 1 in]
        }
        frame "W" {
          w510 = 0.0
          n284 = Unbundle(w507) -> ("Roll"=w502:sgl, "Pitch"=w506:sgl)  [unwired: 2 out]
          n285 = Absolute Value(x=w506) -> (abs(x)=w505:sgl)
          n286 = call "Speed Calculator.vi"("Speed step"=w501, "Previous Speed"=w502) -> ("New Speed"=w503:dbl)
          n287 = call "Speed Calculator.vi"("Speed step"=w501, "Previous Speed"=w505) -> ("New Speed"=w504:dbl)
          n288 = Negate(x=w504) -> (-x=w508:dbl)
          n289 = Bundle("New Speed"=w503, w508, w510, w510) -> (w509:cluster{"New Speed":dbl, dbl, dbl, dbl})  [unwired: 1 in]
        }
        frame "A" {
          w512 = 0.0
          n290 = Bundle(w512, w512, w512, w512) -> (w511:cluster{dbl, dbl, dbl, dbl})  [unwired: 1 in]
        }
        frame Default {
          w517 = 0.0
          n291 = Unbundle(w516) -> ("Roll"=w515:sgl)  [unwired: 3 out]
          n292 = call "Speed Calculator.vi"("Speed step"=w513, "Previous Speed"=w515) -> ("New Speed"=w514:dbl)
          n293 = Bundle("New Speed"=w514, w517, w517, w517) -> (w518:cluster{"New Speed":dbl, dbl, dbl, dbl})  [unwired: 1 in]
        }
      }
    }
    frame "A" {
      # "Switch-case to determine which the second button is."
      n294 = case shown="\"W\"" w521 {
        tunnel: [w532 w543 w554 w565 w575 w586 w589 w598] -> w520
        tunnel: w522 -> [w523 w535 w545 w555 w567 w579 _ w591]
        tunnel: w519 -> [w531 w540 w552 w558 w573 w582 _ w595]
        frame "UP" {
          w528 = 0.0
          n295 = Unbundle(w531) -> ("Roll"=w525:sgl, "Yaw Speed"=w524:sgl)  [unwired: 2 out]
          n296 = Absolute Value(x=w525) -> (abs(x)=w530:sgl)
          n297 = call "Speed Calculator.vi"("Speed step"=w523, "Previous Speed"=w524) -> ("New Speed"=w526:dbl)
          n298 = call "Speed Calculator.vi"("Speed step"=w523, "Previous Speed"=w530) -> ("New Speed"=w529:dbl)
          n299 = Negate(x=w529) -> (-x=w527:dbl)
          n300 = Bundle(w527, w528, "New Speed"=w526, w528) -> (w532:cluster{dbl, dbl, "New Speed":dbl, dbl})  [unwired: 1 in]
        }
        frame "DOWN" {
          w544 = 0.0
          n301 = Unbundle(w540) -> ("Pitch"=w539:sgl, "Vertical Speed"=w538:sgl)  [unwired: 2 out]
          n302 = Absolute Value(x=w539) -> (abs(x)=w536:sgl)
          n303 = Absolute Value(x=w538) -> (abs(x)=w537:sgl)
          n304 = call "Speed Calculator.vi"("Speed step"=w535, "Previous Speed"=w536) -> ("New Speed"=w533:dbl)
          n305 = call "Speed Calculator.vi"("Speed step"=w535, "Previous Speed"=w537) -> ("New Speed"=w534:dbl)
          n306 = Negate(x=w533) -> (-x=w542:dbl)
          n307 = Negate(x=w534) -> (-x=w541:dbl)
          n308 = Bundle(w544, w542, w541, w544) -> (w543:cluster{dbl, dbl, dbl, dbl})  [unwired: 1 in]
        }
        frame "RIGHT" {
          w547 = 0.0
          n309 = Unbundle(w552) -> ("Roll"=w551:sgl, "Yaw Speed"=w546:sgl)  [unwired: 2 out]
          n310 = Absolute Value(x=w551) -> (abs(x)=w550:sgl)
          n311 = call "Speed Calculator.vi"("Speed step"=w545, "Previous Speed"=w546) -> ("New Speed"=w548:dbl)
          n312 = call "Speed Calculator.vi"("Speed step"=w545, "Previous Speed"=w550) -> ("New Speed"=w549:dbl)
          n313 = Negate(x=w549) -> (-x=w553:dbl)
          n314 = Bundle(w553, w547, w547, "New Speed"=w548) -> (w554:cluster{dbl, dbl, dbl, "New Speed":dbl})  [unwired: 1 in]
        }
        frame "LEFT" {
          w564 = 0.0
          n315 = Unbundle(w558) -> ("Roll"=w557:sgl, "Yaw Speed"=w556:sgl)  [unwired: 2 out]
          n316 = Absolute Value(x=w557) -> (abs(x)=w560:sgl)
          n317 = Absolute Value(x=w556) -> (abs(x)=w559:sgl)
          n318 = call "Speed Calculator.vi"("Speed step"=w555, "Previous Speed"=w560) -> ("New Speed"=w562:dbl)
          n319 = call "Speed Calculator.vi"("Speed step"=w555, "Previous Speed"=w559) -> ("New Speed"=w561:dbl)
          n320 = Negate(x=w562) -> (-x=w563:dbl)
          n321 = Negate(x=w561) -> (-x=w566:dbl)
          n322 = Bundle(w563, w564, w564, w566) -> (w565:cluster{dbl, dbl, dbl, dbl})  [unwired: 1 in]
        }
        frame "S" {
          w576 = 0.0
          n323 = Unbundle(w573) -> ("Roll"=w572:sgl, "Pitch"=w569:sgl)  [unwired: 2 out]
          n324 = Absolute Value(x=w572) -> (abs(x)=w571:sgl)
          n325 = call "Speed Calculator.vi"("Speed step"=w567, "Previous Speed"=w569) -> ("New Speed"=w568:dbl)
          n326 = call "Speed Calculator.vi"("Speed step"=w567, "Previous Speed"=w571) -> ("New Speed"=w570:dbl)
          n327 = Negate(x=w570) -> (-x=w574:dbl)
          n328 = Bundle(w574, "New Speed"=w568, w576, w576) -> (w575:cluster{dbl, "New Speed":dbl, dbl, dbl})  [unwired: 1 in]
        }
        frame "W" {
          w587 = 0.0
          n329 = Unbundle(w582) -> ("Roll"=w581:sgl, "Pitch"=w580:sgl)  [unwired: 2 out]
          n330 = Absolute Value(x=w581) -> (abs(x)=w584:sgl)
          n331 = Absolute Value(x=w580) -> (abs(x)=w583:sgl)
          n332 = call "Speed Calculator.vi"("Speed step"=w579, "Previous Speed"=w584) -> ("New Speed"=w577:dbl)
          n333 = call "Speed Calculator.vi"("Speed step"=w579, "Previous Speed"=w583) -> ("New Speed"=w578:dbl)
          n334 = Negate(x=w577) -> (-x=w588:dbl)
          n335 = Negate(x=w578) -> (-x=w585:dbl)
          n336 = Bundle(w588, w585, w587, w587) -> (w586:cluster{dbl, dbl, dbl, dbl})  [unwired: 1 in]
        }
        frame "D" {
          w590 = 0.0
          n337 = Bundle(w590, w590, w590, w590) -> (w589:cluster{dbl, dbl, dbl, dbl})  [unwired: 1 in]
        }
        frame Default {
          w596 = 0.0
          n338 = Unbundle(w595) -> ("Roll"=w594:sgl)  [unwired: 3 out]
          n339 = Absolute Value(x=w594) -> (abs(x)=w593:sgl)
          n340 = call "Speed Calculator.vi"("Speed step"=w591, "Previous Speed"=w593) -> ("New Speed"=w592:dbl)
          n341 = Negate(x=w592) -> (-x=w597:dbl)
          n342 = Bundle(w597, w596, w596, w596) -> (w598:cluster{dbl, dbl, dbl, dbl})  [unwired: 1 in]
        }
      }
    }
    frame Default {
      w600 = 0.0
      n343 = Bundle(w600, w600, w600, w600) -> (w599:cluster{dbl, dbl, dbl, dbl})  [unwired: 1 in]
    }
  }
  "Control Cluster" <- w2
